vi "bead_dropper.vi"() -> ()   [LabVIEW 2014]
panel:
  out "Pulse Number":i32=16
  in  "stop":bool
  out "Current Amplitude (mV)":dbl=13.75
  in  "Amplitude Step (mV)":dbl=0.25
  in  "Start amplitude (mV)":dbl=10.0
  in  "Stop Freq (kHz)":dbl=300.0
  in  "Start Freq (kHz)":dbl=175.0
  in  "Length of pulse (s)":dbl=1.0
  in  "Time betweeen (s)":dbl=4.0
  in  "Number of pulses":u16=40
  # "VI to pulse HP3325a generator (for use with piezo launcher)"
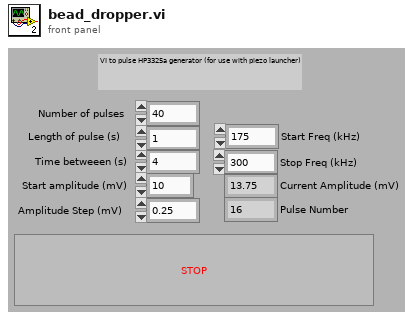
[diagram p1: front panel]
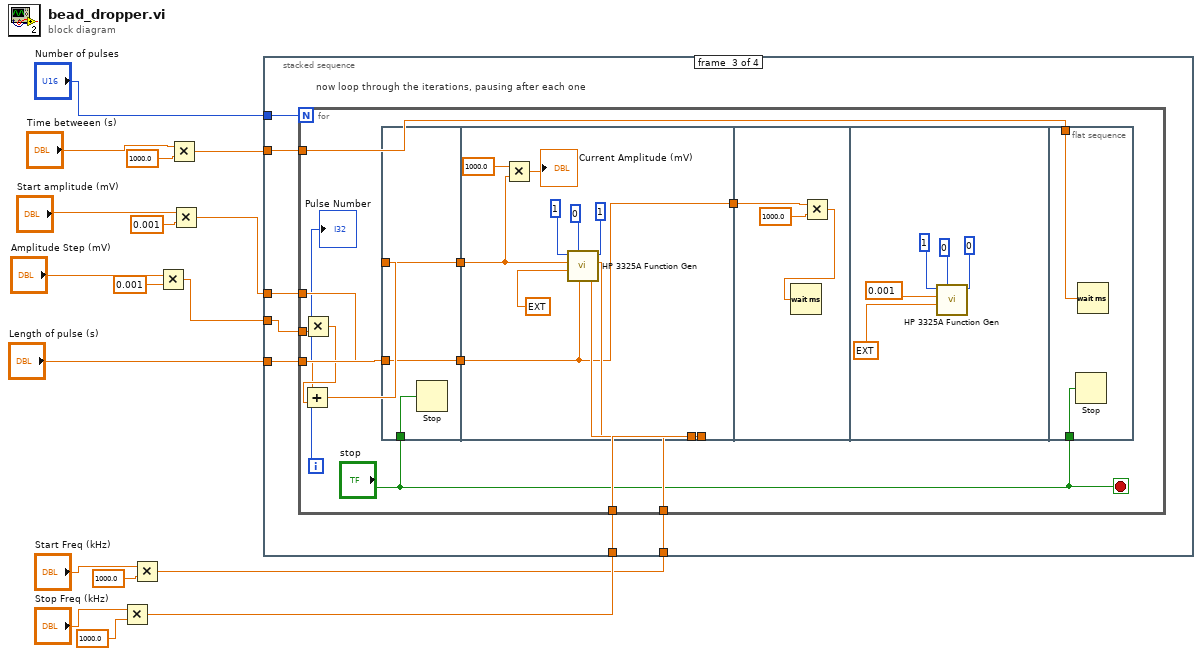
[diagram p0: block diagram]
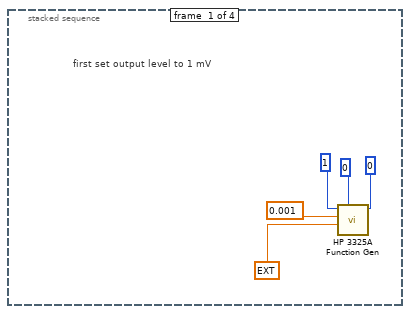
[diagram p2: hidden frame]
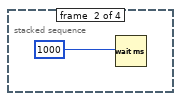
[diagram p3: hidden frame]
diagram:
  n1 = Multiply(x="Stop Freq (kHz)", y=1000.0) -> (x*y=w11:dbl)
  n2 = Multiply(x="Start Freq (kHz)", y=1000.0) -> (x*y=w10:dbl)
  n3 = Multiply(x="Amplitude Step (mV)", y=0.001) -> (x*y=w1:dbl)
  n4 = Multiply(x="Time betweeen (s)", y=1000.0) -> (x*y=w4:dbl)
  n5 = Multiply(x="Start amplitude (mV)", y=0.001) -> (x*y=w7:dbl)
  n6 = stacked-sequence {
    tunnel: "Number of pulses" -> [_ _ w30 _]
    tunnel: w7 -> [_ _ w29 _]
    tunnel: "Length of pulse (s)" -> [_ _ w28 _]
    tunnel: w11 -> [_ _ w27 _]
    tunnel: w10 -> [_ _ w26 _]
    tunnel: w4 -> [_ _ w25 _]
    tunnel: w1 -> [_ _ w24 _]
    frame #0 {
      # "first set output level to 1 mV"
      n7 = call "HP 3325A Function Gen.vi"("sweep function (none:0)"=0, "modulation (off:0)"=0, "offset (V)"=ext 0.0, "amplitude (V)"=0.001, "signal type (dc:0)"=i16 1) -> ()  [unwired: 5 in]
    }
    frame #1 {
      n8 = Wait (ms)(milliseconds to wait=1000) -> ()  [unwired: 1 out]
    }
    frame #2 {
      # "now loop through the iterations, pausing after each one"
      n9 = for {
        N: w30 -> [_]
        tunnel: w29 -> [w36]
        tunnel: w28 -> [w38]
        tunnel: w27 -> [w43]
        tunnel: w26 -> [w42]
        tunnel: w25 -> [w41]
        tunnel: w24 -> [w39]
        i -> [w34]
        stop <- "stop" stop-if-true
        n10 = Multiply(x=w34, y=w39) -> (x*y=w37:dbl)
        n11 = Add(x=w36, y=w37) -> (x+y=w35:dbl)
        n12 = flat-sequence {
          tunnel: w35 -> [w45]
          tunnel: w38 -> [w46]
          tunnel: [w46] -> w33
          tunnel: [w45] -> w32
          tunnel: "stop" -> [w44]
          tunnel: w43 -> [w53]
          tunnel: w42 -> [w52]
          tunnel: [w50] -> w40
          tunnel: w33 -> [w50]
          tunnel: w32 -> [w48]
          tunnel: w40 -> [w58]
          tunnel: w41 -> [w66]
          tunnel: "stop" -> [w65]
          frame #0 {
            n13 = Stop(stop? (T)=w44) -> ()
          }
          frame #1 {
            n14 = Multiply(x=1000.0, y=w48) -> (x*y=→"Current Amplitude (mV)":dbl)
            n15 = call "HP 3325A Function Gen.vi"("stop"=w53, "start"=w52, "sweep function (none:0)"=1, "sweep time (S)"=w50, "modulation (off:0)"=0, "offset (V)"=ext 0.0, "amplitude (V)"=w48, "signal type (dc:0)"=i16 1) -> ()  [unwired: 2 in]
          }
          frame #2 {
            n16 = Multiply(x=w58, y=1000.0) -> (x*y=w57:dbl)
            n17 = Wait (ms)(milliseconds to wait=w57) -> ()  [unwired: 1 out]
          }
          frame #3 {
            n18 = call "HP 3325A Function Gen.vi"("sweep function (none:0)"=0, "modulation (off:0)"=0, "offset (V)"=ext 0.0, "amplitude (V)"=0.001, "signal type (dc:0)"=i16 1) -> ()  [unwired: 5 in]
          }
          frame #4 {
            n19 = Stop(stop? (T)=w65) -> ()
            n20 = Wait (ms)(milliseconds to wait=w66) -> ()  [unwired: 1 out]
          }
        }
        "Pulse Number" <- w34
      }
    }
    frame #3 {
    }
  }
